vi "Tren_Masas.vi"() -> ()   [LabVIEW 2017]
uses:
  <vilib>/addons/Control Design/_Model Construction/Data Typedefs.llb/CD Variables.ctl
  <vilib>/Simulation/Scripting/Companion Diagram/SimConfigNode/SimParams.ctl
  <vilib>/Simulation/Scripting/Companion Diagram/SimConfigNode/_simSolvers.ctl
  <vilib>/Simulation/Implementation/Shared/SIMSCR Execution Mode.ctl
  <vilib>/Simulation/Param Hierarchy/Typedefs/SIMPH Param Control Actions.ctl
  <vilib>/Simulation/Implementation/Shared/NILVSim_ParamChanged.vi
  <vilib>/Simulation/Implementation/Shared/NILVSIM_BeginStep.vi
  <vilib>/Simulation/DataSources/Implementation/NILVSim Step.llb/SIM Step (vector).vi
  <vilib>/Simulation/Utility/Implementation/SIM Halt.vi
  <vilib>/Simulation/DataSources/Implementation/NILVSim Sine Wave.llb/SIM Sine Wave (vector).vi
  <vilib>/Simulation/ContinuousLinear/Implementation/NILVSim State Space.llb/SIM State Space Distributor (CD).vi
  <vilib>/Simulation/ContinuousLinear/Implementation/NILVSim State Space.llb/SIM State Space Collector (CD).vi
  <vilib>/Simulation/SignalDisplay/Implementation/NILVSim Time Waveform.llb/SIM Time Waveform (vector).vi
  <vilib>/Simulation/Implementation/Shared/NILVSim_Manager.vi
  <vilib>/Utility/error.llb/Clear Errors.vi
  <vilib>/Simulation/Implementation/Shared/NILVSim_FinalizeModel.vi
  <vilib>/addons/Control Design/_Model Construction/Model Creation.llb/Model Creation SubVI/cd_Create Symbolic State Space Model.vi
  <vilib>/addons/Control Design/_Utility/Model Viewer.llb/Model Viewer SubVI/cd_Draw State-Space Equation (SS).vi
  <vilib>/picture/3D Picture Control/Object/Create Object (drawable).vi
  <vilib>/Simulation/Implementation/Shared/SIM Unbundle Sim Info.vi
  <vilib>/Simulation/Implementation/Shared/NILVSim_Initialize.vi
  <vilib>/picture/3D Picture Control/Object/Find Object.vi
  <vilib>/picture/3D Picture Control/Transformations/Set Translation.vi
  <vilib>/picture/3D Picture Control/Object/Add Object.vi
  <vilib>/picture/3D Picture Control/Object/Add Object (reference).vi
  <vilib>/Simulation/Utility/Implementation/NILVSim Get Time and IsAcceptedStep.vi
  <vilib>/Simulation/Implementation/Shared/SIMSH Read Queue.vi
  <vilib>/Simulation/Implementation/Shared/NILVSim_GetModelError.vi
  <vilib>/Simulation/Implementation/Shared/SIM Bundle Sim Info.vi
  <vilib>/Simulation/Scripting/Companion Diagram/SimConfigNode/SimDog.xnode
  <vilib>/Simulation/Implementation/XNodeFramework/SimXNode/SimX.xnode
  <vilib>/addons/Control Design/_Model Construction/Model Typedefs.llb/CD General Elements.ctl
  <vilib>/addons/Control Design/_Model Construction/NI_LinSys_Model Typedefs.lvlib
  <vilib>/addons/Control Design/_Model Construction/Model Typedefs.llb/CD State Space Model (MIMO).ctl
  <vilib>/addons/Control Design/_Model Construction/NI_LinSys_Model Creation.lvlib
  <vilib>/addons/Control Design/_Utility/NI_CD_Model Viewer.lvlib
  <vilib>/picture/3D Picture Control/NI_3D Picture Control.lvlib
  <vilib>/Simulation/ContinuousLinear/Implementation/NILVSim State Space.llb/SIM State Space (CD).vi
  <vilib>/Simulation/Implementation/Shared/NI_SIM_Implementation.lvlib
  <vilib>/addons/Control Design/_Model Construction/NI_LinSys_Data Typedefs.lvlib
panel:
  in  "s":bool
  out "3D Picture":refnum<vi>(3d-picture)
  out "Equation":picture
  in  "Variables":T1=[{"Name"="k1", " Value"=1.0}, {"Name"="k2", " Value"=1.0}, {"Name"="k3", " Value"=1.0}, {"Name"="b1", " Value"=1.0}, {"Name"="b2", " Value"=1.0}, {"Name"="b3", " Value"=1.0}, {"Name"="m1", " Value"=1.0}, {"Name"="m2", " Value"=1.0}, {"Name"="m3", " Value"=1.0}] {"Value" format="%.2f"}
  in  "Halt?":bool
  out "Waveform Chart":waveform(dbl)[](graph)
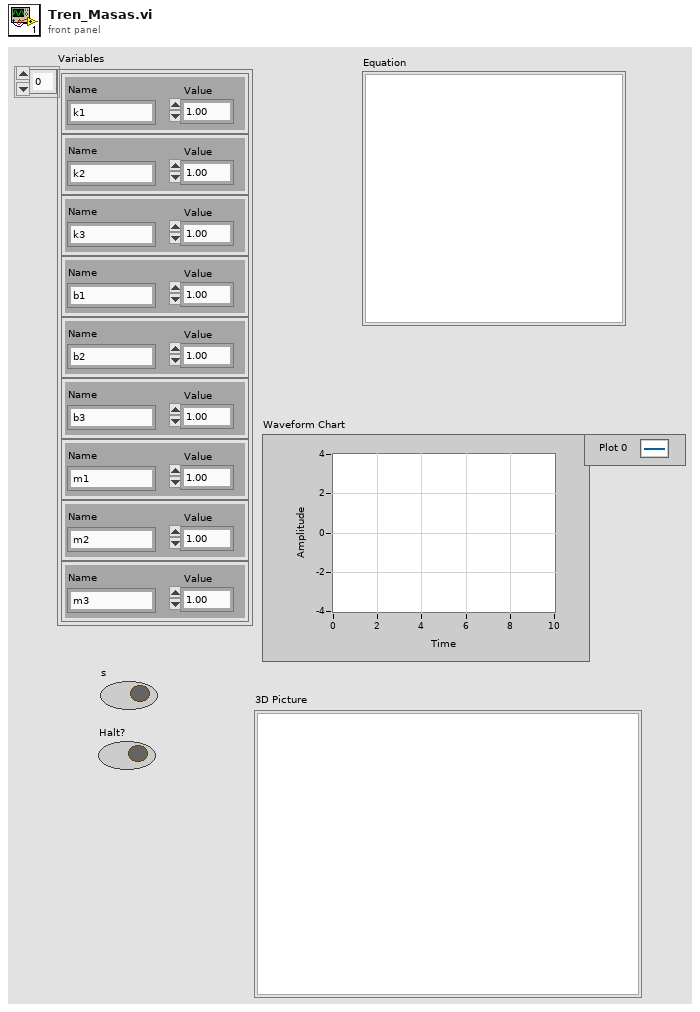
[diagram p1: front panel]
types:
  T1 = typedef "NI_LinSys_Data Typedefs.lvlib/CD Variables.ctl" = cluster{"Name":string, " Value":dbl}[]
  T2 = cluster{"Red":sgl, "Green":sgl, "Blue":sgl, "Alpha":sgl}
  T3 = typedef "NI_LinSys_Model Typedefs.lvlib/CD State Space Model (MIMO).ctl" = cluster{"properties":T4, "A":dbl[][], "B":dbl[][], "C":dbl[][], "D":dbl[][], "StateNames":string[], "Transport Delay":dbl[][]}
  T4 = typedef "NI_LinSys_Model Typedefs.lvlib/CD General Elements.ctl" = cluster{"Model name":string, "Input names":string[], "Output names":string[], "Input Delays":dbl[], "Output Delays":dbl[], "Sampling Time":dbl, "Notes":string}
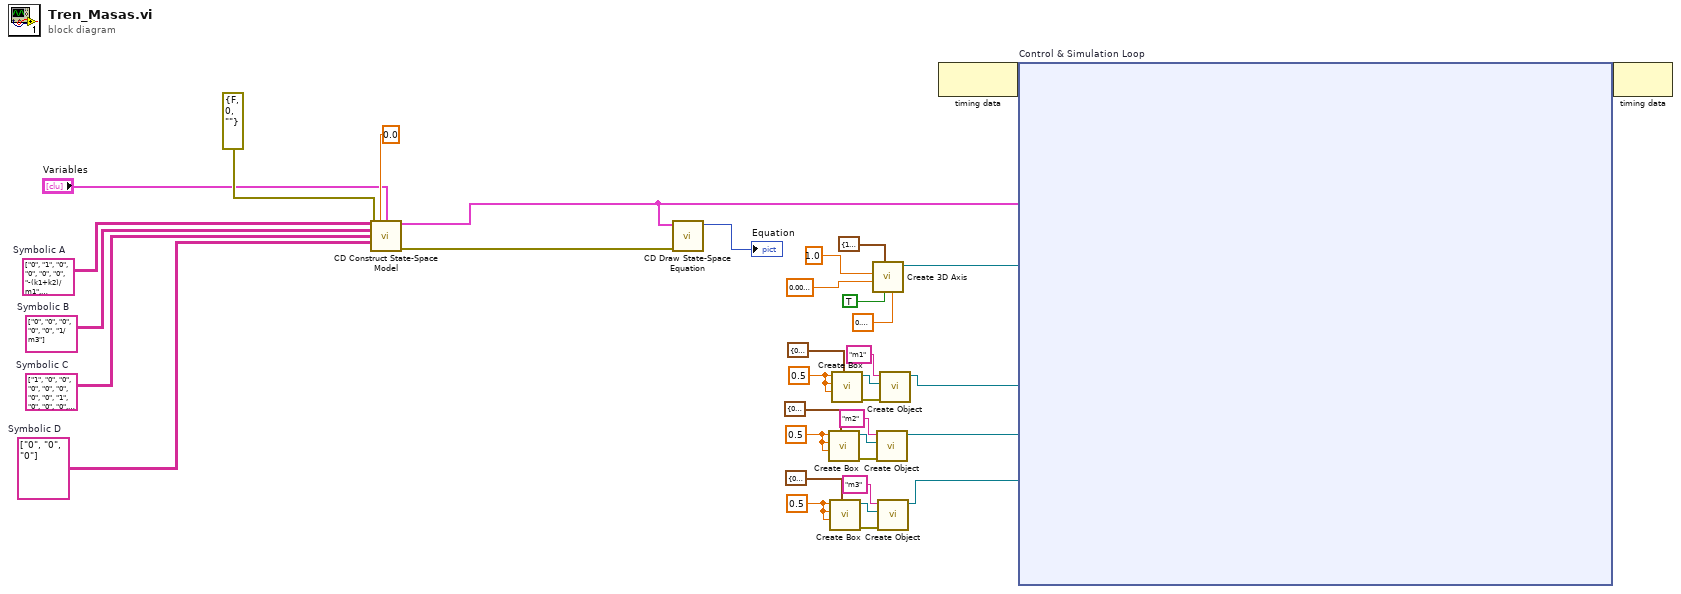
[diagram p0: block diagram]
diagram:
  w11 = sgl 0.5 ("Length X")
  w12 = sgl 0.5 ("Length X")
  w24 = sgl 0.5 ("Length X")
  w25 = string[][] [["0"], ["0"], ["0"]]  # Symbolic D
  w26 = string[][] [["1", "0", "0", "0", "0", "0"], ["0", "0", "1", "0", "0", "0"], ["0", "0", "0", "0", "1", "0"]]  # Symbolic C
  w27 = string[][] [["0"], ["0"], ["0"], ["0"], ["0"], ["1/m3"]]  # Symbolic B
  w28 = string[][] [["0", "1", "0", "0", "0", "0"], ["-(k1+k2)/m1", "-(b1+b2)/m1", "k2/m1", "b2/m1", "0", "0"], ["0", "0", "0", "1", "0", "0"], ["k2/m2", "b2/m2", "-(k2+k3)/m2", "-(b2+b3)/m2", "k3/m2", "b3/m2"], ["0", "0", "0", "0", "0", "1"], ["0", "0", "k3/m3", "b3/m3", "-k3/m3", "-b3/m3"]]  # Symbolic A
  n1 = call-poly <vilib>:"CD Construct State-Space Model.vi"("Symbolic A"=w28, "Sampling Time (s)"=0.0, "Symbolic B"=w27, "Symbolic C"=w26, "Symbolic D"=w25, "error in (no error)"=errorcluster {"status"=FALSE, "code"=0, "source"=""}, "Variables"="Variables") -> ("State Space Model"=w31:T3, "error out"=w30:errorcluster)  [unwired: 7 in]
  n2 = call-poly <vilib>:"CD Draw State-Space Equation.vi"("error in (no error)"=w30, "State-Space Model"=w31) -> ("Equation"=→"Equation":picture)  [unwired: 7 in, 2 out]
  n3 = call <vilib>:"Create Box.vi"("Color"=T2 {"Red"=0.0, "Green"=1.0, "Blue"=0.0, "Alpha"=1.0}, "Length Z"=w12, "Length Y"=w12, "Length X"=w12) -> ("error out"=w14:errorcluster, "New Box Refnum"=w15:refnum<vi>)  [unwired: 6 in]
  n4 = call <vilib>:"Create Box.vi"("Color"=T2 {"Red"=0.0, "Green"=1.0, "Blue"=0.0, "Alpha"=1.0}, "Length Z"=w11, "Length Y"=w11, "Length X"=w11) -> ("error out"=w9:errorcluster, "New Box Refnum"=w8:refnum<vi>)  [unwired: 6 in]
  n5 = call <vilib>:"Create Box.vi"("Color"=T2 {"Red"=0.0, "Green"=1.0, "Blue"=0.0, "Alpha"=1.0}, "Length Z"=w24, "Length Y"=w24, "Length X"=w24) -> ("error out"=w22:errorcluster, "New Box Refnum"=w21:refnum<vi>)  [unwired: 6 in]
  n6 = call <vilib>:"Create 3D Axis.vi"("Character Size"=sgl 0.1, "Axis label?"=TRUE, "Color"=T2 {"Red"=1.0, "Green"=0.0, "Blue"=0.0, "Alpha"=1.0}, "Radius"=sgl 0.01, "Length"=sgl 1.0) -> ("New Object Refnum"=w1:refnum<vi>)  [unwired: 5 in, 1 out]
  n7 = call-poly <vilib>:"Create Object.vi"("error in (no error)"=w14, "Geometry"=w15, "Name"="m2") -> ("Scene:New Object"=w7:refnum<vi>)  [unwired: 7 in, 1 out]
  n8 = call-poly <vilib>:"Create Object.vi"("error in (no error)"=w9, "Geometry"=w8, "Name"="m3") -> ("Scene:New Object"=w6:refnum<vi>)  [unwired: 7 in, 1 out]
  n9 = call-poly <vilib>:"Create Object.vi"("error in (no error)"=w22, "Geometry"=w21, "Name"="m1") -> ("Scene:New Object"=w2:refnum<vi>)  [unwired: 7 in, 1 out]
  n10 = node-c288() -> (w36:variant)  [unwired: 1 in]
  n11 = node-c254 "Control & Simulation Loop"(w36, w31, w1, w2, w7, w6) -> (w35:variant)
  n12 = node-c288(w35) -> ()  [unwired: 1 out]
